vi "Write Search.vi"(10 "Search":refnum<class "Search.lvclass">, 11 "DiagramObject in":refnum<class "DiagramObject.lvclass">) -> (3 "DiagramObject out":refnum<class "DiagramObject.lvclass">)   [LabVIEW 2016, in "DiagramObject.lvclass"]
uses:
  DiagramObject.lvclass
  Search/Search.lvclass
  DiagramObject.lvclass/DiagramObject.ctl
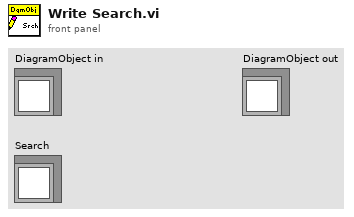
[diagram p1: front panel]
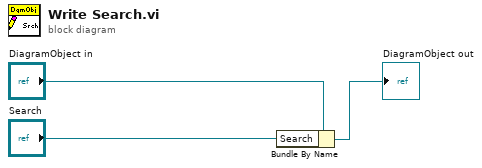
[diagram p0: block diagram]
diagram:
  n1 = Bundle By Name(cluster="DiagramObject in", "Search"="Search") -> (→"DiagramObject out":refnum<class "DiagramObject.lvclass">)
